vi "Initialize OAuth for GitLab.vi"(6 "Refresh Token":string, 7 "Authorization Server URI":string, 9 "GitLab Access Scope":T1={"api"=FALSE, "read_user"=TRUE, "read_api"=TRUE, "read_repository"=TRUE, "write_repository"=FALSE, "read_registry"=FALSE, "write_registry"=FALSE, "sudo"=FALSE, "openid"=FALSE, "profile"=FALSE, "email"=FALSE}, 10 "Client Secret":string, 11 "Client ID":string) -> (0 "error out":errorcluster, 3 "Oauth2.GitLab":refnum<class "Oauth2.GitLab.lvclass">)   [LabVIEW 2013, in "Oauth2.GitLab.lvclass"]
uses:
  Oauth2.GitLab.lvclass
  GitLab Access Scope -- cluster.ctl
  Oauth2/Oauth2.lvclass
  <vilib>/LabVIEW Open Source Project/Data Manipulation/Variant/OpenVariant.lvlib
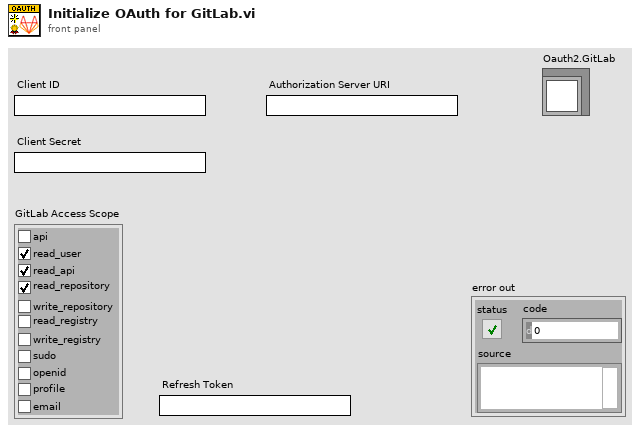
[diagram p1: front panel]
types:
  T1 = typedef "Oauth2.GitLab.lvclass/GitLab Access Scope -- cluster.ctl" = cluster{"api":bool, "read_user":bool, "read_api":bool, "read_repository":bool, "write_repository":bool, "read_registry":bool, "write_registry":bool, "sudo":bool, "openid":bool, "profile":bool, "email":bool}
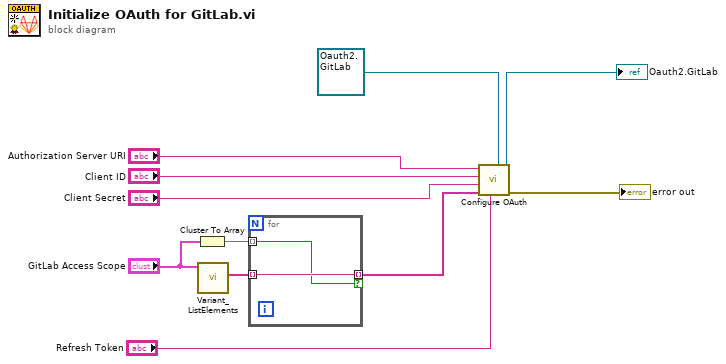
[diagram p0: block diagram]
diagram:
  n1 = Cluster To Array(cluster="GitLab Access Scope") -> (array=w5:bool[])
  n2 = call <vilib>:"Variant_ListElements.vi"("Variant"="GitLab Access Scope") -> ("element names"=w6:string[])  [unwired: 7 in, 3 out]
  n3 = for {
    tunnel: [w13] -> w3 mode=indexing if=w12
    tunnel: w6 -> [w13] mode=indexing
    tunnel: w5 -> [w12] mode=indexing
  }
  n4 = call "Configure OAuth.vi"("Oauth2 in"=refnum<class "Oauth2.GitLab.lvclass"> refnum ("Oauth2.GitHub in"), "Refresh Token"="Refresh Token", "scopes"=w3, "Client Secret"="Client Secret", "Client ID"="Client ID", "Authorization Server URI"="Authorization Server URI") -> ("error out"=→"error out":errorcluster, "Oauth2"=→"Oauth2.GitLab":refnum<class "Oauth2.GitLab.lvclass">)  [unwired: 4 in]
